vi "ShhgCommandCenter.vi"() -> ()   [LabVIEW 2015]
doc: "This template is for the Queued Message Handler design pattern.\n\nThe Event Handling Loop generates messages based on user interface actions.\n\nThe Message Handling Loop processes messages generated by the Event Handling Loop, or by other messages. The messages are string values, so new messages can be added easily to the Message Cases case structure in the Message Handling Loop. Each message cluster can also provide an optional value for Message Data, which is a variant that can be converted to whatever message-specific data is required."
uses:
  NetworkStream/NetworkStreamData.ctl
  ShhgDataLogging/DataLoggingCluster.ctl
  controls/UI Data.ctl
  DeviceLoopData.ctl
  DeviceState.ctl
  <vilib>/dex/Stream Element Allocation Mode.ctl
  <vilib>/dex/Flush And Wait Empty Condition.ctl
  <vilib>/Utility/error.llb/DialogType.ctl
  <vilib>/Utility/error.llb/Error Cluster From Error Code.vi
  support/Message Queue/Enqueue Message (Single).vi
  support/Message Queue/Enqueue Message (Array).vi
  <vilib>/ErrorRing/Error Ring.xnode
  support/Message Queue/Message Queue.lvlib
  support/User Events/User Events.lvlib
  support/Error Handling/Error Handling.lvlib
  NetworkStream/NetworkStream.lvlib
  ShhgDataLogging/ShhgDataLogging.lvlib
panel:
  out "Waiting for devices":bool
  out "Shots to go...":i32
  in  "Randomize":bool
  in  "AbortShooting":bool
  in  "Shoot":bool
  in  "RequestStatusAllDevices":bool
  in  "DisconnectAllDevices":bool
  in  "Next Shot Number":u32
  in  "Target Tabs":enum32{"Target", "Configuration"}(tab)
  out "Waiting after shot":bool
  out "Target Sequence Length (ms)":dbl=100.0
  out "Target up to date":bool
  out "Target Ready":bool
  out "Target Status":string
  out "Target Connected":bool caption="Connected"
  in  "Sequence Length (ms)":dbl=100.0
  in  "Abort Waiting after shot":bool
  in  "TargetReaderURL":string="//localhost:SolidTargetSequenceControl/SolidTargetSequenceControl"
  in  "TargetNetworkSharedVariable":refnum<k21>="ni.var.psp://localhost/SolidTargetSequenceControl/Status"
  in  "Logging Tabs":enum32{"Data Logging", "Configuration"}(tab)
  in  "DataLoggingCluster":T1={"Shot No. "=0, "Pulse Energy (mJ)"=0.0, "Pulse Duration (fs)"=0.0, "Chirp (fs^2)"=0.0, "Wedge Insertion (mm)"=0.0, "Parabola Position (um)"=0.0, "Delay (ps)"=0.0, "Seq. Length (ms)"=100.0, "Add. Param. No 1"=0.0, "Add. Param. No 2"=0.0, "Notes"=""} {"Add. Param. No 2" format="%#_6f"; "Add. Param. No 1" format="%#_6f"; "Wedge Insertion (mm)" format="%#_6f"; "Pulse Duration (fs)" format="%#_6f"; "Parabola Position (um)" format="%#_6f"; "Pulse Energy (mJ)" format="%#_6f"; "Chirp (fs^2)" format="%#_6f"}
  in  "Experiment Folder Path":path
  in  "ConnectAllDevices":bool
  out "Loop Active":bool caption="Active"
  in  "Abort Loop":bool
  in  "DelayLineTabs":enum32{"DelayLine", "Configuration"}(tab)
  out "DelayLine up to date":bool
  out "DelayLine Ready":bool
  in  "DelayLine Setpoint (ps)":dbl
  out "Delay":dbl
  out "DelayLineStatus":string
  out "DelayLineConnected":bool caption="Connected"
  in  "DelayLineReaderURL":string="//192.168.178.65/DelayLine"
  in  "DelayLineNetworkSharedVariable":refnum<k21>="ni.var.psp://pc-loa231/DelayLine/Status"
  in  "Loop End":dbl
  in  "Loop Stepsize":dbl=1.0
  in  "Loop Start":dbl
  in  "Loop Over":T2(ring)
  in  "Start Loop":bool
  in  "Exit":bool
  # "USED BY TARGET"
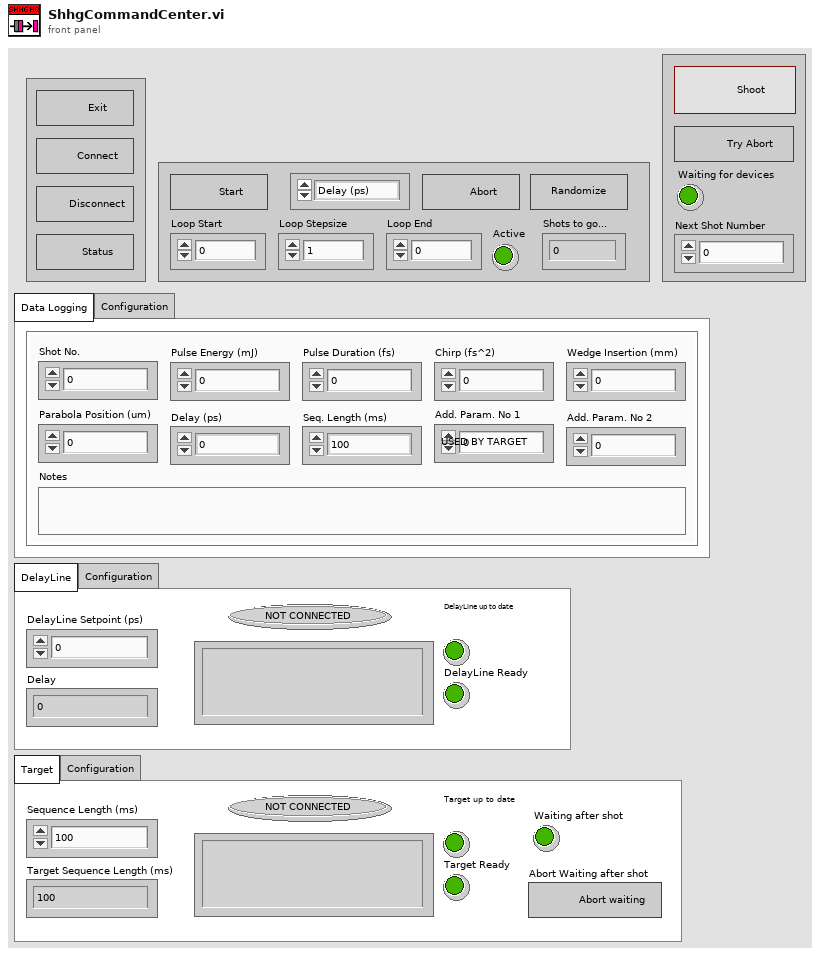
[diagram p1: front panel]
types:
  T1 = typedef "ShhgDataLogging.lvlib/DataLoggingCluster.ctl" = cluster{"Shot No. ":u32, "Pulse Energy (mJ)":dbl, "Pulse Duration (fs)":dbl, "Chirp (fs^2)":dbl, "Wedge Insertion (mm)":dbl, "Parabola Position (um)":dbl, "Delay (ps)":dbl, "Seq. Length (ms)":dbl, "Add. Param. No 1":dbl, "Add. Param. No 2":dbl, "Notes":string}
  T2 = enum16{"Delay (ps)", "Wedge (mm)", "Chirp (fs²)"}
  T3 = typedef "DeviceState.ctl" = enum16{"NotConnected", "Connected"}
  T4 = typedef "DeviceLoopData.ctl" = cluster{"shared variable refnum":refnum<k21>, "Hash":u64, "writer endpoint":refnum<k21>, "Sequence Number":u64}
  T5 = typedef "UI Data.ctl" = cluster{"Boolean <Replace Me>":bool, "String <Replace Me>":string, "Numeric <Replace Me>":dbl, "Do Something Ref":refnum<vi>, "Do Something Else Ref":refnum<vi>, "Data Display Ref":refnum<vi>, "Exit Button Ref":refnum<vi>, "LoopArray":dbl[]}
  T6 = typedef "User Events.lvlib/User Events.ctl" = cluster{"Stop":refnum<user-event>, "UserEventNo2":refnum<user-event>}
  T7 = typedef "Message Queue.lvlib/All Message Queues.ctl" = cluster{"UI":refnum<queue>, "DelayLine":refnum<queue>, "Target":refnum<queue>, "Logging":refnum<queue>}
  T8 = typedef "DialogType.ctl" = u16
  T9 = typedef "NetworkStream.lvlib/NetworkStreamData.ctl" = cluster{"Command/Status":string, "Data":variant, "Session Hash":u64, "Sequence Number":u64}
  T10 = typedef "Stream Element Allocation Mode.ctl" = u32
  T11 = typedef "Flush And Wait Empty Condition.ctl" = u8
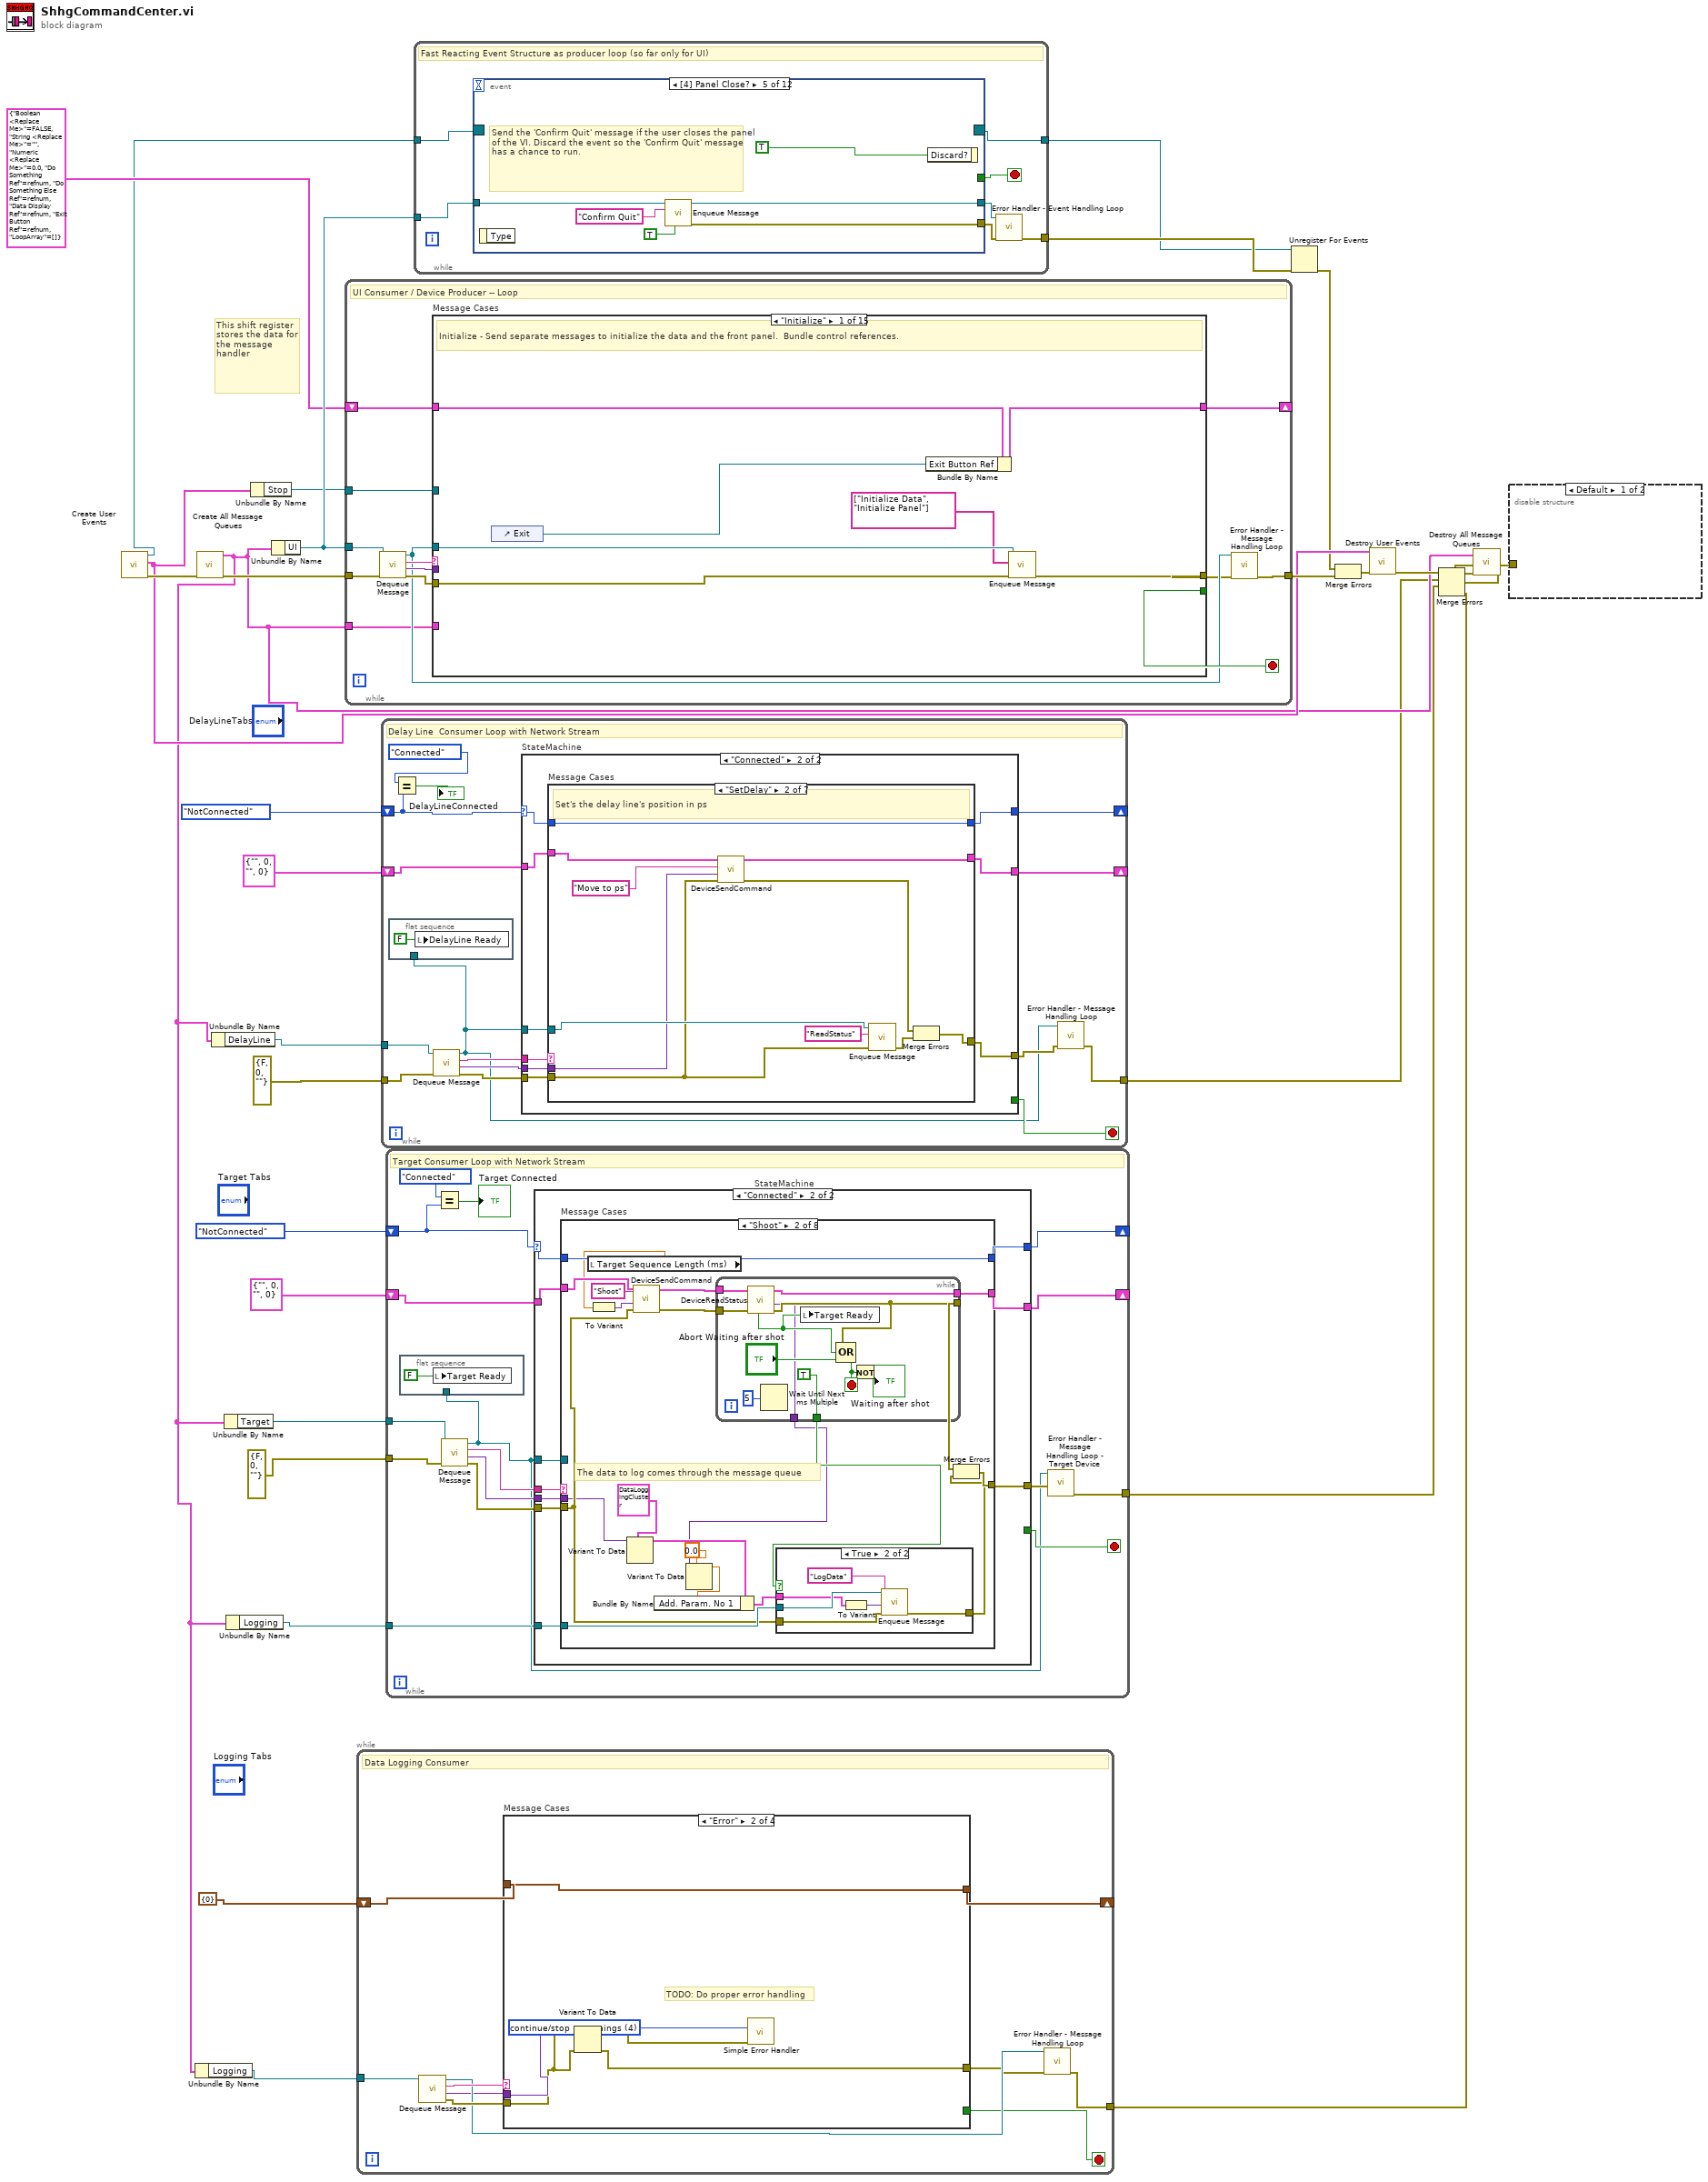
[diagram p0: block diagram]
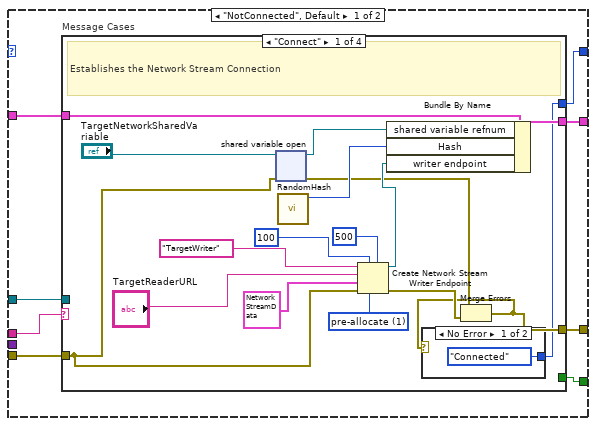
[diagram p2: hidden frame]
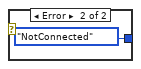
[diagram p3: hidden frame]
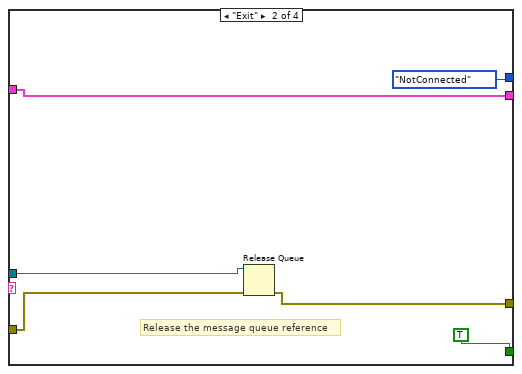
[diagram p4: hidden frame]
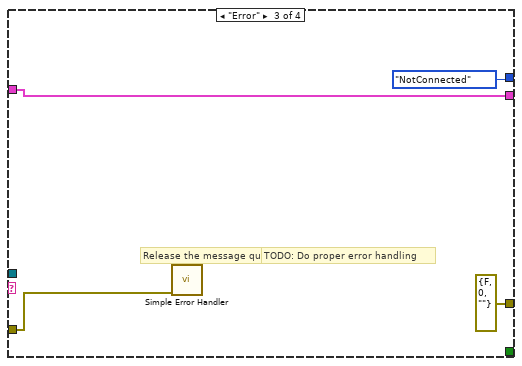
[diagram p5: hidden frame]
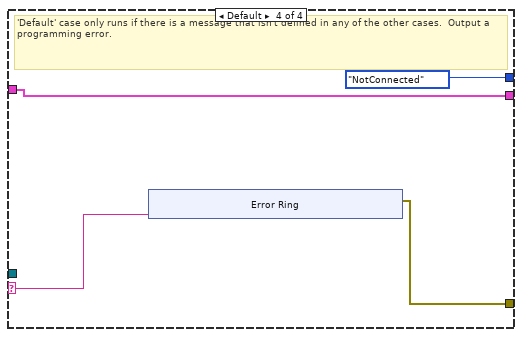
[diagram p6: hidden frame]
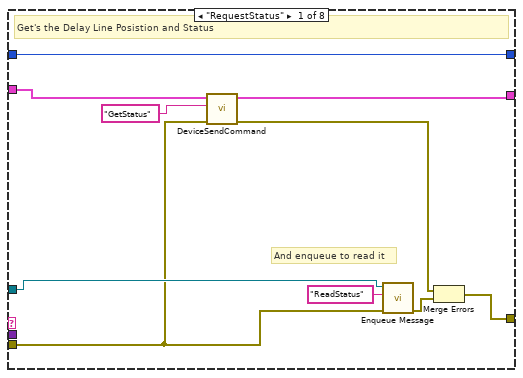
[diagram p7: hidden frame]
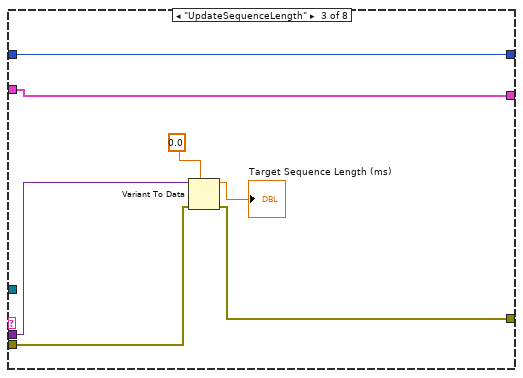
[diagram p9: hidden frame]
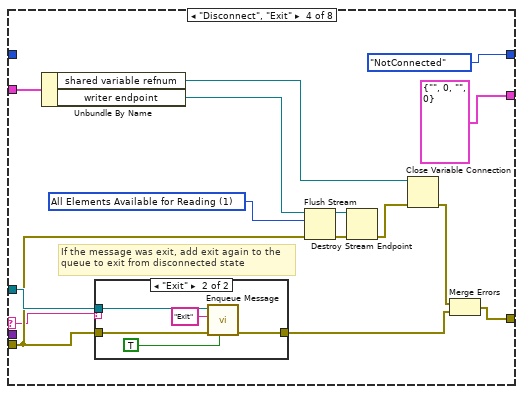
[diagram p10: hidden frame]
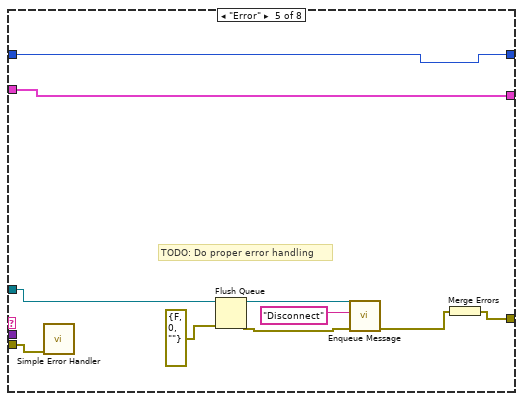
[diagram p12: hidden frame]
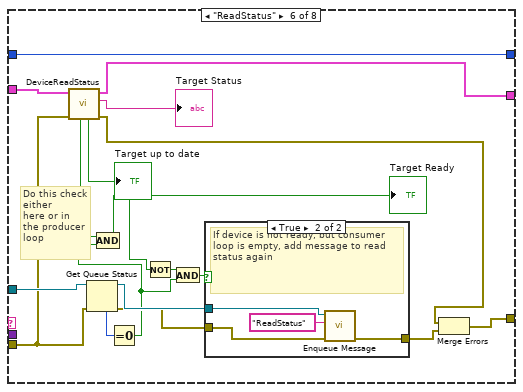
[diagram p13: hidden frame]
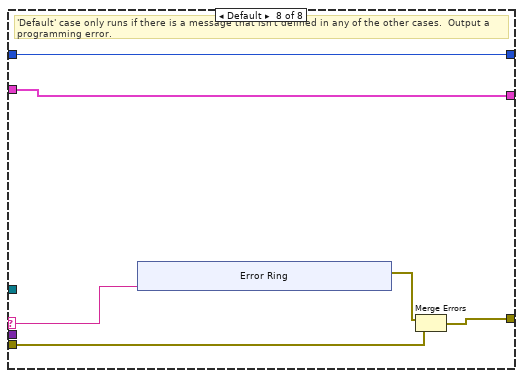
[diagram p16: hidden frame]
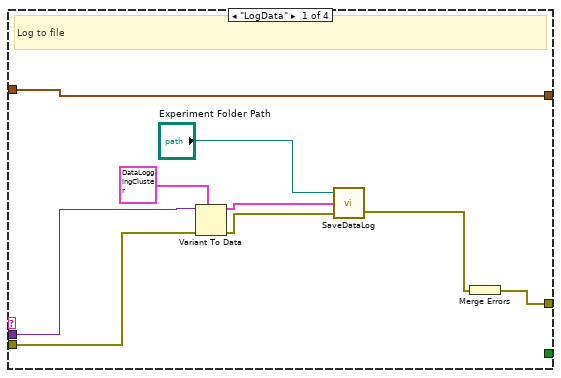
[diagram p17: hidden frame]
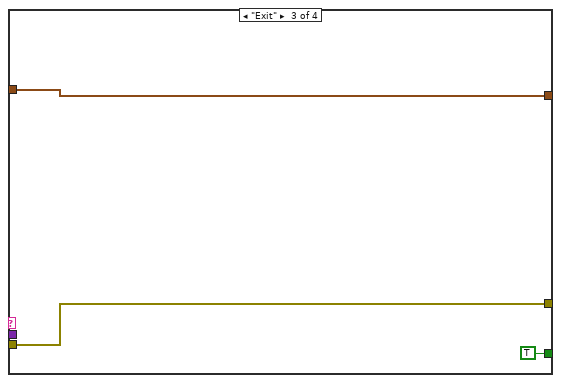
[diagram p18: hidden frame]
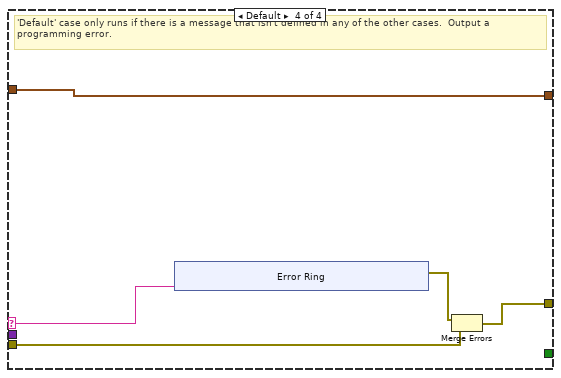
[diagram p19: hidden frame]
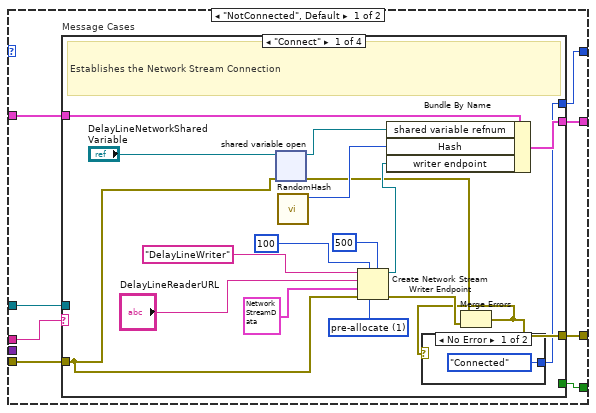
[diagram p20: hidden frame]
diagram:
  # "This shift register stores the data for the message handler"
  n1 = call "Create User Events.vi"() -> ("error out"=w27:errorcluster, "User Events"=w25:T6, "User Events Registration Refnum"=w16:refnum<event-registration>)  [unwired: 9 in]
  n2 = call "Create All Message Queues.vi"("error in (no error)"=w27) -> ("error out"=w30:errorcluster, "Message Queues out"=w6:T7)  [unwired: 9 in]
  n3 = Unbundle By Name(w6) -> ("Logging"=w13:refnum<queue>)
  n4 = Unbundle By Name(w6) -> ("DelayLine"=w18:refnum<queue>)
  n5 = Unbundle By Name(w6) -> ("Target"=w12:refnum<queue>)
  n6 = Unbundle By Name(w6) -> ("Logging"=w8:refnum<queue>)
  n7 = Unbundle By Name(w25) -> ("Stop"=w14:refnum<user-event>)
  n8 = Unbundle By Name(w6) -> ("UI"=w28:refnum<queue>)
  n9 = while {
    tunnel: w28 -> [w35]
    shift-right: [w42] -> _
    shift-left: T5 {"Boolean <Replace Me>"=FALSE, "String <Replace Me>"="", "Numeric <Replace Me>"=0.0, "Do Something Ref"=refnum, "Do Something Else Ref"=refnum, "Data Display Ref"=refnum, "Exit Button Ref"=refnum, "LoopArray"=[]} ("Data Cluster") -> [w43]
    tunnel: w14 -> [w40]
    tunnel: w30 -> [w39]
    tunnel: [w33] -> w29
    tunnel: w6 -> [w31]
    stop <- w41 stop-if-true
    # "UI Consumer / Device Producer -- Loop"
    n10 = call "Dequeue Message.vi"("error in (no error)"=w39, "Message Queue"=w35) -> ("error out"=w38:errorcluster, "Message Data"=w36:variant, "Message"=w37:string, "dup Message Queue"=w34:refnum<queue>)  [unwired: 6 in]
    n11 = case "Message Cases" shown="\"Initialize\"" w37 {
      selector: w37 -> [_ _ _ _ _ w95 _ _ _ _ _ _ _ _ w254]
      tunnel: w34 -> [w48 _ w57 w69 w81 _ _ w136 w154 _ _ _ _ w253 _]
      tunnel: w38 -> [w49 w55 w58 w77 w85 w97 w110 w138 w152 w205 w215 w225 w235 w246 _]
      tunnel: [w50 w51 w59 w70 w83 w98 w107 w137 w150 w202 w216 w226 w236 w249 w255] -> w32
      tunnel: w43 -> [w47 w54 w60 w76 w84 w99 w116 w145 w153 w207 w217 w227 w237 w252 w256]
      tunnel: [w46 w53 w60 w76 w84 w99 w116 w144 w155 w207 w217 w227 w237 w252 w256] -> w42
      tunnel: [_ _ _ _ _ _ _ _ _ _ _ _ _ TRUE _] -> w41
      tunnel: w36 -> [_ _ _ w75 _ w96 _ _ _ w200 _ _ _ _ _]
      tunnel: w40 -> [_ _ _ _ _ _ _ _ _ _ _ _ _ w248 _]
      tunnel: w31 -> [_ _ _ _ _ w93 w115 _ w151 w204 w210 w220 w230 w242 _]
      frame "Initialize" {
        # "Initialize - Send separate messages to initialize the data and the front panel.  Bundle control references."
        n12 = control-ref of="Exit"() -> (w45:refnum<vi>)
        n13 = Bundle By Name(cluster=w47, "Exit Button Ref"=w45) -> (w46:T5)
        n14 = call-poly "Enqueue Message.vi"("error in (no error)"=w49, "Message Array"=string[] ["Initialize Data", "Initialize Panel"], "Message Queue"=w48) -> ("error out"=w50:errorcluster)  [unwired: 7 in, 1 out]
      }
      frame "Initialize Data" {
        # "#CodeNeeded - Initialize your state data here."
        # "Initialize Data - Initialize the state data cluster."
        n15 = Bundle By Name(cluster=w54, "String <Replace Me>"="Initial Message" ("Initial Message")) -> (w53:T5)
        n16 = Merge Errors(w55) -> (w51:errorcluster)
      }
      frame "Initialize Panel" {
        # "Initialize Panel - Initialize the appearance of the front panel here."
        n17 = disable-structure shown="Disabled" {
          disable-tunnel: w60 -> [w66 _]
          disable-tunnel: w58 -> [w65 _]
          disable-tunnel: w57 -> [w64 _]
          disable-tunnel: [w63 _] -> w56
          frame Disabled {
            # "Send string to \"Update Display\" message"
            # "#CodeNeeded - Initialize the appearance of the front panel"
            n18 = Unbundle By Name(w66) -> ("String <Replace Me>"=w61:string)
            n19 = call-poly "Enqueue Message.vi"("error in (no error)"=w65, "Message Data"=w61, "Message"="Update Display", "Message Queue"=w64) -> ("error out"=w63:errorcluster)  [unwired: 6 in, 1 out]
          }
          frame Enabled {
          }
        }
        n20 = Merge Errors(w56) -> (w59:errorcluster)
      }
      frame "Error" {
        # "#CodeRecommended - If you ever change the name of this \"Error\" message, you'll need to update the name in the Check Loop Error.vi as well."
        # "#CodeRecommended - This code will always pop up an error dialog and call the 'Exit' message if an error occurs. Add more fine-grained error handling here."
        # "Error - Check the error message data and respond accordingly. This message is sent by the \"Error Handler\" VIs at the end of each loop in this application."
        n21 = Variant To Data(error in=w77, type=errorcluster {"status"=FALSE, "code"=0, "source"=""} ("error constant"), Variant=w75) -> (data=w73:errorcluster, error out=w72:errorcluster)
        n22 = call <vilib>:"Simple Error Handler.vi"("error in (no error)"=w73) -> ()  [unwired: 4 in, 5 out]
        n23 = call-poly "Enqueue Message.vi"("Priority Message? (F)"=TRUE, "Message"="Exit", "Message Queue"=w69) -> ("error out"=w71:errorcluster)  [unwired: 7 in, 1 out]
        n24 = Merge Errors(w71, w72) -> (w70:errorcluster)
      }
      frame "Confirm Quit" {
        # "#CodeNeeded - If you want to provide an \"Are you sure\" dialog (or some other notification) before the application exits, place that code here. This message is typically sent from a Panel Close? event."
        # "Confirm Quit - Message that can confirm whether or not the user wants to exit the application."
        n25 = Two Button Dialog(message="Do you really want to quit?", 2:"Yes!" ("T button name (\"OK\")")) -> (T button?=w78:bool)  [unwired: 1 in]
        n26 = case shown="False" w78 {
          tunnel: w85 -> [w86 w91]
          tunnel: [w86 w90] -> w82
          tunnel: w81 -> [_ w89]
          frame False {
          }
          frame True {
            n27 = call-poly "Enqueue Message.vi"("Priority Message? (F)"=TRUE, "error in (no error)"=w91, "Message"="Exit", "Message Queue"=w89) -> ("error out"=w90:errorcluster)  [unwired: 6 in, 1 out]
          }
        }
        n28 = Merge Errors(w82) -> (w83:errorcluster)
      }
      frame "SetDelay" {
        # "Duplicate this frame when creating new messages.  Change this comment in the duplicated frame to describe this message."
        n29 = Unbundle By Name(w93) -> ("DelayLine"=w92:refnum<queue>)
        n30 = call-poly "Enqueue Message.vi"("error in (no error)"=w97, "Message Data"=w96, "Message"=w95, "Message Queue"=w92) -> ("error out"=w94:errorcluster)  [unwired: 6 in, 1 out]
        n31 = Merge Errors(w94) -> (w98:errorcluster)
      }
      frame "Shoot" {
        # "Actually if the last status was ready, there should be no reason why they are not ready anmore."
        # "wait some time for target to get busy, TODO: or wait for 'Target Ready' variable to turn false"
        n32 = Unbundle By Name(w115) -> ("DelayLine"=w112:refnum<queue>, "Target"=w111:refnum<queue>)
        n33 = Increment(x="Next Shot Number") -> (x+1=w114:u32)
        n34 = local write "Next Shot Number"(w114) -> ()
        n35 = call-poly "Enqueue Message.vi"("error in (no error)"=w110, "Message"="RequestStatus", "Message Queue"=w112) -> ("error out"=w103:errorcluster)  [unwired: 7 in, 1 out]
        n36 = call-poly "Enqueue Message.vi"("error in (no error)"=w103, "Message"="RequestStatus", "Message Queue"=w111) -> ("error out"=w102:errorcluster, "dup Message Queue"=w109:refnum<queue>)  [unwired: 7 in]
        n37 = property on="Shot No." class="DigNum (strict)"(error in=w102, "Value"="Next Shot Number") -> (error out=w101:errorcluster)  [unwired: 1 in, 1 out]
        n38 = while {
          tunnel: ["AbortShooting"] -> w108
          tunnel: [w126] -> w100
          tunnel: w101 -> [w126]
          stop <- w128 stop-if-true
          n39 = local read "DelayLine Ready"() -> (w133:bool)
          n40 = local read "Target Ready"() -> (w132:bool)
          n41 = And(x=w133, y=w132) -> (x .and. y?=w131:bool)
          n42 = Or(x=w131, y="AbortShooting") -> (x .or. y?=w128:bool)
          n43 = Not(x=w128) -> (.not. x?=→"Waiting for devices":bool)
          n44 = Wait Until Next ms Multiple(millisecond multiple=u32 5) -> ()  [unwired: 1 out]
        }
        n45 = case shown="False" w108 {
          tunnel: [w120 w125] -> w107
          tunnel: w109 -> [w122 _]
          tunnel: w100 -> [w121 w125]
          tunnel: [200 0] -> w106
          frame False {
            n46 = To Variant(anything="DataLoggingCluster") -> (Variant=w118:variant)
            n47 = call-poly "Enqueue Message.vi"("error in (no error)"=w121, "Message Data"=w118, "Message"="Shoot", "Message Queue"=w122) -> ("error out"=w120:errorcluster)  [unwired: 6 in, 1 out]
          }
          frame True {
          }
        }
        n48 = Wait (ms)(milliseconds to wait=w106) -> ()  [unwired: 1 out]
      }
      frame "Start Loop" {
        # "This just generates the loop array and then dispatches the continue loop message"
        n49 = call-poly "Enqueue Message.vi"("error in (no error)"=w138, "Message"="Continue Loop", "Message Queue"=w136) -> ("error out"=w137:errorcluster)  [unwired: 7 in, 1 out]
        n50 = call "CreateLoopArray.vi"("Randomize"="Randomize", "Loop Stepsize"="Loop Stepsize", "Loop End"="Loop End", "Loop Start"="Loop Start") -> ("Loop Array"=w143:dbl[])  [unwired: 7 in]
        n51 = Bundle By Name(cluster=w145, "LoopArray"=w143) -> (w144:T5)
        n52 = local write "Loop Active"(TRUE ("Loop Active")) -> ()
      }
      frame "Continue Loop" {
        # "This just generates the loop array and then dispatches the continue loop message"
        n53 = Unbundle By Name(w153) -> ("LoopArray"=w149:dbl[])
        n54 = Array Size(array=w149) -> (size(s)=w147:i32)
        "Shots to go..." <- w147
        n55 = Not Equal To 0?(x=w147) -> (x != 0?=w148:bool)
        n56 = case shown="True" w148 {
          tunnel: [w158 w173] -> w155
          tunnel: w154 -> [_ w172]
          tunnel: w153 -> [w158 w171]
          tunnel: w149 -> [_ w170]
          tunnel: w152 -> [w156 w167]
          tunnel: w151 -> [_ w165]
          tunnel: [w156 w162] -> w150
          tunnel: [FALSE w159] -> w146
          frame False {
          }
          frame True {
            n57 = while "Wait for the target to finish shooting" {
              tunnel: ["Abort Loop"] -> w160
              tunnel: w167 -> [w193]
              tunnel: [w193] -> w164
              stop <- w195 stop-if-true
              n58 = local read "Target Ready"() -> (w196:bool)
              n59 = Or(x="Abort Loop", y=w196) -> (x .or. y?=w195:bool)
              n60 = Wait Until Next ms Multiple(millisecond multiple=u32 5) -> ()  [unwired: 1 out]
            }
            n61 = Delete From Array(array=w170, index=0) -> (deleted portion=w163:dbl, array with subset deleted=w169:dbl[])  [unwired: 1 in]
            n62 = case "Set the parameter" shown="\"Delay (ps)\", Default" "Loop Over" {
              tunnel: w165 -> [w189 _]
              tunnel: w164 -> [w190 w191]
              tunnel: w163 -> [w187 _]
              tunnel: [w184 w191] -> w161
              frame "Delay (ps)", Default {
                n63 = Unbundle By Name(w189) -> ("DelayLine"=w188:refnum<queue>)
                n64 = To Variant(anything=w187) -> (Variant=w186:variant)
                n65 = call-poly "Enqueue Message.vi"("error in (no error)"=w190, "Message Data"=w186, "Message"="SetDelay", "Message Queue"=w188) -> ("error out"=w184:errorcluster)  [unwired: 6 in, 1 out]
              }
              frame "Wedge (mm)" {
              }
            }
            n66 = Bundle By Name(cluster=w171, "LoopArray"=w169) -> (w173:T5)
            n67 = case "Enqueue continuation" shown="True" w160 {
              tunnel: w172 -> [w181 _]
              tunnel: [w177 w183] -> w162
              tunnel: w161 -> [w175 w183]
              tunnel: [TRUE FALSE] -> w159
              frame False {
                n68 = call-poly "Enqueue Message.vi"("error in (no error)"=w175, "Message"="Shoot", "Message Queue"=w181) -> ("error out"=w179:errorcluster, "dup Message Queue"=w178:refnum<queue>)  [unwired: 7 in]
                n69 = call-poly "Enqueue Message.vi"("error in (no error)"=w179, "Message"="Continue Loop", "Message Queue"=w178) -> ("error out"=w177:errorcluster)  [unwired: 7 in, 1 out]
              }
              frame True {
              }
            }
          }
        }
        "Loop Active" <- w146
      }
      frame "UpdateSequenceLength" {
        n70 = Unbundle By Name(w204) -> ("Target"=w203:refnum<queue>)
        n71 = call-poly "Enqueue Message.vi"("error in (no error)"=w205, "Message Data"=w200, "Message"="UpdateSequenceLength", "Message Queue"=w203) -> ("error out"=w198:errorcluster)  [unwired: 6 in, 1 out]
        n72 = Variant To Data(error in=w198, type=0.0 ("Value"), Variant=w200) -> (data=w199:dbl, error out=w197:errorcluster)
        n73 = property on="Seq. Length (ms)" class="DigNum (strict)"(error in=w197, "Value"=w199) -> (error out=w202:errorcluster)  [unwired: 1 in, 1 out]
      }
      frame "ConnectAllDevices" {
        # "Duplicate this frame when creating new messages.  Change this comment in the duplicated frame to describe this message."
        n74 = Unbundle By Name(w210) -> ("DelayLine"=w209:refnum<queue>, "Target"=w208:refnum<queue>)
        n75 = call-poly "Enqueue Message.vi"("error in (no error)"=w215, "Message"="Connect", "Message Queue"=w208) -> ("error out"=w211:errorcluster)  [unwired: 7 in, 1 out]
        n76 = call-poly "Enqueue Message.vi"("error in (no error)"=w211, "Message"="Connect", "Message Queue"=w209) -> ("error out"=w212:errorcluster)  [unwired: 7 in, 1 out]
        n77 = Merge Errors(w212) -> (w216:errorcluster)
      }
      frame "DisconnectAllDevices" {
        # "Duplicate this frame when creating new messages.  Change this comment in the duplicated frame to describe this message."
        n78 = Unbundle By Name(w220) -> ("DelayLine"=w219:refnum<queue>, "Target"=w218:refnum<queue>)
        n79 = call-poly "Enqueue Message.vi"("error in (no error)"=w225, "Message"="Disconnect", "Message Queue"=w218) -> ("error out"=w221:errorcluster)  [unwired: 7 in, 1 out]
        n80 = call-poly "Enqueue Message.vi"("error in (no error)"=w221, "Message"="Disconnect", "Message Queue"=w219) -> ("error out"=w222:errorcluster)  [unwired: 7 in, 1 out]
        n81 = Merge Errors(w222) -> (w226:errorcluster)
      }
      frame "RequestStatusAllDevices" {
        # "Duplicate this frame when creating new messages.  Change this comment in the duplicated frame to describe this message."
        n82 = Unbundle By Name(w230) -> ("DelayLine"=w229:refnum<queue>, "Target"=w228:refnum<queue>)
        n83 = call-poly "Enqueue Message.vi"("error in (no error)"=w235, "Message"="RequestStatus", "Message Queue"=w228) -> ("error out"=w231:errorcluster)  [unwired: 7 in, 1 out]
        n84 = call-poly "Enqueue Message.vi"("error in (no error)"=w231, "Message"="RequestStatus", "Message Queue"=w229) -> ("error out"=w232:errorcluster)  [unwired: 7 in, 1 out]
        n85 = Merge Errors(w232) -> (w236:errorcluster)
      }
      frame "Exit" {
        w241 = "Exit" ("Message")
        w243 = TRUE ("Priority Message? (F)")
        # "Stop the VI"
        # "Release the message queue reference"
        # "#CodeNeeded - Add any required cleanup code here"
        # "Exit - Exit the application."
        n86 = Unbundle By Name(w242) -> ("DelayLine"=w240:refnum<queue>, "Logging"=w239:refnum<queue>, "Target"=w238:refnum<queue>)
        n87 = call-poly "Enqueue Message.vi"("Priority Message? (F)"=w243, "error in (no error)"=w246, "Message"=w241, "Message Queue"=w238) -> ("error out"=w245:errorcluster)  [unwired: 6 in, 1 out]
        n88 = call "Fire User Event - Stop.vi"("User Event - Stop"=w248) -> ("error out"=w247:errorcluster)  [unwired: 10 in]
        n89 = Release Queue(queue=w253, error in (no error)=w246) -> (error out=w250:errorcluster)  [unwired: 1 in, 2 out]
        n90 = call-poly "Enqueue Message.vi"("Priority Message? (F)"=w243, "error in (no error)"=w245, "Message"=w241, "Message Queue"=w239) -> ("error out"=w244:errorcluster)  [unwired: 6 in, 1 out]
        n91 = call-poly "Enqueue Message.vi"("Message"=w241, "Message Queue"=w240) -> ()  [unwired: 8 in, 2 out]
        n92 = Merge Errors(w247, w250, w244) -> (w249:errorcluster)
      }
      frame Default {
        # "'Default' case only runs if there is a message that isn't defined in any of the other cases.  Output a programming error."
        n93 = xnode "Error Ring"("parameter 0"=w254) -> ("error out"=w255:errorcluster)
      }
    }
    n94 = call "Error Handler - Message Handling Loop.vi"("error in (no error)"=w32, "Message Queue"=w34) -> ("dup error in"=w33:errorcluster)  [unwired: 8 in, 1 out]
  }
  n95 = while {
    shift-right: [w272] -> _
    shift-left: cluster{i32} {0} -> [w271]
    tunnel: w13 -> [w265]
    tunnel: [w267] -> w1
    stop <- w264 stop-if-true
    # "Data Logging Consumer"
    n96 = call "Dequeue Message.vi"("Message Queue"=w265) -> ("error out"=w270:errorcluster, "Message Data"=w266:variant, "Message"=w273:string, "dup Message Queue"=w269:refnum<queue>)  [unwired: 7 in]
    n97 = case "Message Cases" shown="\"Error\"" w273 {
      selector: w273 -> [_ _ _ w296]
      tunnel: [w281 w288 w289 w295] -> w272
      tunnel: w271 -> [w281 w288 w289 w295]
      tunnel: w270 -> [w277 w285 w290 w294]
      tunnel: [w282 w286 w290 w293] -> w268
      tunnel: w266 -> [w280 w287 _ _]
      tunnel: [_ _ TRUE _] -> w264
      frame "LogData" {
        # "Log to file"
        n98 = Variant To Data(error in=w277, type=T1 {"Shot No. "=0, "Pulse Energy (mJ)"=0.0, "Pulse Duration (fs)"=0.0, "Chirp (fs^2)"=0.0, "Wedge Insertion (mm)"=0.0, "Parabola Position (um)"=0.0, "Delay (ps)"=0.0, "Seq. Length (ms)"=0.0, "Add. Param. No 1"=0.0, "Add. Param. No 2"=0.0, "Notes"=""} ("DataLoggingCluster"), Variant=w280) -> (data=w278:T1, error out=w275:errorcluster)
        n99 = call "SaveDataLog.vi"("entrée d'erreur"=w275, "DataLoggingCluster"=w278, "chemin du fichier (utiliser une boîte de dialogue)"="Experiment Folder Path") -> ("sortie d'erreur"=w274:errorcluster)  [unwired: 1 in]
        n100 = Merge Errors(w274) -> (w282:errorcluster)
      }
      frame "Error" {
        w283 = T8 4 items=["no dialog", "OK message", "continue or stop message", "OK message + warnings", "continue/stop + warnings"] ("type of dialog (OK msg:1)")
        # "TODO: Do proper error handling"
        n101 = Variant To Data(error in=w285, type=w285, Variant=w287) -> (data=w284:errorcluster, error out=w286:errorcluster)
        n102 = call <vilib>:"Simple Error Handler.vi"("type of dialog (OK msg:1)"=w283, "error in (no error)"=w284) -> ()  [unwired: 3 in, 5 out]
      }
      frame "Exit" {
      }
      frame Default {
        # "'Default' case only runs if there is a message that isn't defined in any of the other cases.  Output a programming error."
        n103 = xnode "Error Ring"("parameter 0"=w296) -> ("error out"=w292:errorcluster)
        n104 = Merge Errors(w292, w294) -> (w293:errorcluster)
      }
    }
    n105 = call "Error Handler - Message Handling Loop.vi"("error in (no error)"=w268, "Message Queue"=w269) -> ("dup error in"=w267:errorcluster)  [unwired: 8 in, 1 out]
  }
  n106 = while {
    shift-right: [w318] -> _
    shift-left: DeviceState."NotConnected" -> [w315]
    shift-right: [w313] -> _
    shift-left: T4 {"shared variable refnum"="", "Hash"=0, "writer endpoint"="", "Sequence Number"=0} -> [w312]
    tunnel: w18 -> [w307]
    tunnel: errorcluster {"status"=FALSE, "code"=0, "source"=""} ("error in (no error)") -> [w311]
    tunnel: [w308] -> w3
    stop <- w305 stop-if-true
    # "Delay Line  Consumer Loop with Network Stream"
    n107 = flat-sequence {
      tunnel: w304 -> [_]
      frame #0 {
        n108 = local write "DelayLine Ready"(FALSE ("DelayLine Ready")) -> ()
      }
    }
    n109 = Equal?(x=DeviceState."Connected", y=w315) -> (x = y?=→"DelayLineConnected":bool)
    n110 = call "Dequeue Message.vi"("error in (no error)"=w311, "Message Queue"=w307) -> ("error out"=w310:errorcluster, "Message Data"=w306:variant, "Message"=w317:string, "dup Message Queue"=w304:refnum<queue>)  [unwired: 6 in]
    n111 = case "StateMachine" shown="\"Connected\"" w315 {
      selector: w315 -> [_ w373]
      tunnel: [w322 w372] -> w318
      tunnel: w317 -> [w327 w375]
      tunnel: [w326 w370] -> w313
      tunnel: w312 -> [w325 w376]
      tunnel: w310 -> [w324 w374]
      tunnel: [w323 w371] -> w309
      tunnel: w304 -> [w321 w369]
      tunnel: w306 -> [_ w368]
      tunnel: [w320 _] -> w305
      frame "NotConnected", Default {
        n112 = case "Message Cases" shown="\"Connect\"" w327 {
          selector: w327 -> [_ _ _ w360]
          tunnel: [w344 w347 w355 w359] -> w326
          tunnel: w325 -> [w343 w347 w355 w359]
          tunnel: w324 -> [w333 w352 w354 _]
          tunnel: [w329 w350 errorcluster {"status"=FALSE, "code"=0, "source"=""} ("error out") w357] -> w323
          tunnel: [w328 DeviceState."NotConnected" DeviceState."NotConnected" DeviceState."NotConnected"] -> w322
          tunnel: w321 -> [_ w351 _ _]
          tunnel: [_ TRUE _ _] -> w320
          frame "Connect" {
            w337 = T10 1 items=["allocate as needed", "pre-allocate"] ("element allocation mode")
            # "Establishes the Network Stream Connection"
            n113 = shared-variable-open("DelayLineNetworkSharedVariable", w333) -> (w341:refnum<k21>, w331:errorcluster)
            n114 = call "RandomHash.vi"() -> ("Numeric Control"=w340:u64)  [unwired: 11 in]
            n115 = Create Network Stream Writer Endpoint(5:500 ("timeout in ms (-1)"), 6:w337, 7:100 ("writer buffer size"), 8:w333, 9:T9 {"Command/Status"="", "Data"=variant, "Session Hash"=0, "Sequence Number"=0} ("NetworkStreamCluster"), 10:"DelayLineReaderURL", 11:"DelayLineWriter" ("writer name")) -> (0:w330:errorcluster, 3:w332:refnum<k21>)
            n116 = Bundle By Name(cluster=w343, "shared variable refnum"=w341, "Hash"=w340, "writer endpoint"=w332) -> (w344:T4)
            n117 = Merge Errors(w331, w330) -> (w329:errorcluster)
            n118 = case shown="No Error" w329 {
              tunnel: [DeviceState."Connected" ("x") DeviceState."NotConnected"] -> w328
              frame No Error {
              }
              frame Error {
              }
            }
          }
          frame "Exit" {
            # "Release the message queue reference"
            n119 = Release Queue(queue=w351, error in (no error)=w352) -> (error out=w350:errorcluster)  [unwired: 1 in, 2 out]
          }
          frame "Error" {
            # "TODO: Do proper error handling"
            # "Release the message queue reference"
            n120 = call <vilib>:"Simple Error Handler.vi"("error in (no error)"=w354) -> ()  [unwired: 4 in, 5 out]
          }
          frame Default {
            # "'Default' case only runs if there is a message that isn't defined in any of the other cases.  Output a programming error."
            n121 = xnode "Error Ring"("parameter 0"=w360) -> ("error out"=w357:errorcluster)
          }
        }
      }
      frame "Connected" {
        n122 = case "Message Cases" shown="\"SetDelay\"" w375 {
          selector: w375 -> [_ _ w398 _ _ _ w468]
          tunnel: [w383 w394 T4 {"shared variable refnum"="", "Hash"=0, "writer endpoint"="", "Sequence Number"=0} w424 w448 w462 w467] -> w370
          tunnel: w376 -> [w385 w396 w407 w424 w449 w462 w467]
          tunnel: w374 -> [w378 w389 w401 w420 w443 w460 w465]
          tunnel: [w377 w388 w400 w428 w441 w460 w464] -> w371
          tunnel: w373 -> [w386 w397 _ w425 w445 w461 w466]
          tunnel: [w386 w397 DeviceState."NotConnected" w425 w445 w461 w466] -> w372
          tunnel: w369 -> [w381 w392 w402 w423 w444 _ _]
          tunnel: w368 -> [_ w387 _ _ _ _ _]
          frame "RequestStatus" {
            # "Get's the Delay Line Posistion and Status"
            n123 = call "DeviceSendCommand.vi"("error in (no error)"=w378, "Command/Status"="GetStatus", "DeviceLoopData"=w385) -> ("error out"=w379:errorcluster, "DeviceLoopData Out"=w383:T4)  [unwired: 7 in]
            n124 = call-poly "Enqueue Message.vi"("error in (no error)"=w378, "Message"="ReadStatus", "Message Queue"=w381) -> ("error out"=w380:errorcluster)  [unwired: 7 in, 1 out]
            n125 = Merge Errors(w379, w380) -> (w377:errorcluster)
          }
          frame "SetDelay" {
            # "Set's the delay line's position in ps"
            n126 = call "DeviceSendCommand.vi"("error in (no error)"=w389, "Data"=w387, "Command/Status"="Move to ps", "DeviceLoopData"=w396) -> ("error out"=w390:errorcluster, "DeviceLoopData Out"=w394:T4)  [unwired: 6 in]
            n127 = call-poly "Enqueue Message.vi"("error in (no error)"=w389, "Message"="ReadStatus", "Message Queue"=w392) -> ("error out"=w391:errorcluster)  [unwired: 7 in, 1 out]
            n128 = Merge Errors(w390, w391) -> (w388:errorcluster)
          }
          frame "Disconnect", "Exit" {
            w412 = T11 1 items=["All Elements Read From Stream", "All Elements Available for Reading"] ("wait condition")
            # "If the message was exit, add exit again to the\nqueue to exit from disconnected state"
            n129 = Unbundle By Name(w407) -> ("shared variable refnum"=w408:refnum<k21>, "writer endpoint"=w406:refnum<k21>)
            n130 = case shown="\"Exit\"" w398 {
              tunnel: w402 -> [_ w416]
              tunnel: w401 -> [w413 w415]
              tunnel: [w413 w414] -> w399
              frame "False", Default {
              }
              frame "Exit" {
                n131 = call-poly "Enqueue Message.vi"("Priority Message? (F)"=TRUE, "error in (no error)"=w415, "Message"="Exit", "Message Queue"=w416) -> ("error out"=w414:errorcluster)  [unwired: 6 in, 1 out]
              }
            }
            n132 = Flush Stream(8:w401, 10:w412, 11:w406) -> (0:w411:errorcluster, 3:w410:refnum<k21>)  [unwired: 1 in, 1 out]
            n133 = Destroy Stream Endpoint(8:w411, 11:w410) -> (0:w404:errorcluster)
            n134 = Close Variable Connection(8:w404, 11:w408) -> (0:w403:errorcluster)
            n135 = Merge Errors(w403, w399) -> (w400:errorcluster)
          }
          frame "Error" {
            # "TODO: Do proper error handling"
            n136 = call <vilib>:"Simple Error Handler.vi"("error in (no error)"=w420) -> ()  [unwired: 4 in, 5 out]
            n137 = Flush Queue(queue=w423, error in (no error)=errorcluster {"status"=FALSE, "code"=0, "source"=""}) -> (queue out=w422:refnum<queue>, error out=w421:errorcluster)  [unwired: 1 out]
            n138 = call-poly "Enqueue Message.vi"("error in (no error)"=w421, "Message"="Disconnect", "Message Queue"=w422) -> ("error out"=w427:errorcluster)  [unwired: 7 in, 1 out]
            n139 = Merge Errors(w427) -> (w428:errorcluster)
          }
          frame "ReadStatus" {
            # "Do this check either\nhere or in the producer loop"
            n140 = call "DeviceReadStatus.vi"("error in (no error)"=w443, "DeviceLoopData in"=w449) -> ("error out"=w450:errorcluster, "Data"=w451:variant, "Status"=→"DelayLineStatus":string, "DeviceLoopData out"=w448:T4, "Up To Date"=→"DelayLine up to date":bool, "Ready"=w440:bool)  [unwired: 4 in]
            n141 = Get Queue Status(queue=w444, error in (no error)=w443) -> (queue out=w433:refnum<queue>, error out=w434:errorcluster, # elements in queue=w442:i32)  [unwired: 1 in, 5 out]
            n142 = Equal To 0?(x=w442) -> (x = 0?=w435:bool)
            n143 = Compound Arithmetic op=AND(w440, w435) -> (w436:bool)
            n144 = Not(x=w436) -> (.not. x?=w438:bool)
            n145 = Variant To Data(error in=w450, type=0.0, Variant=w451) -> (data=w431:dbl, error out=w432:errorcluster)
            "Delay" <- w431
            n146 = And(x=w438, y=w435) -> (x .and. y?=w437:bool)
            n147 = case shown="False" w437 {
              tunnel: w433 -> [_ w459]
              tunnel: w434 -> [w455 w458]
              tunnel: [w455 w457] -> w439
              frame False {
              }
              frame True {
                # "If device is not ready, but consumer loop is empty, add message to read status again"
                n148 = call-poly "Enqueue Message.vi"("error in (no error)"=w458, "Message"="ReadStatus", "Message Queue"=w459) -> ("error out"=w457:errorcluster)  [unwired: 7 in, 1 out]
              }
            }
            n149 = property on="Delay (ps)" class="DigNum (strict)"(error in=w432, "Value"=w431) -> (error out=w430:errorcluster)  [unwired: 1 in, 1 out]
            n150 = flat-sequence {
              tunnel: w436 -> [w454]
              tunnel: w430 -> [w453]
              tunnel: [w453] -> w429
              frame #0 {
                # "Only be ready when also the data has been written"
                "DelayLine Ready" <- w454
              }
            }
            n151 = Merge Errors(w429, w439) -> (w441:errorcluster)
          }
          frame "Connect" {
            # "Nothing to do here"
          }
          frame Default {
            # "'Default' case only runs if there is a message that isn't defined in any of the other cases.  Output a programming error."
            n152 = xnode "Error Ring"("parameter 0"=w468) -> ("error out"=w463:errorcluster)
            n153 = Merge Errors(w463, w465) -> (w464:errorcluster)
          }
        }
      }
    }
    n154 = call "Error Handler - Message Handling Loop.vi"("error in (no error)"=w309, "Message Queue"=w304) -> ("dup error in"=w308:errorcluster)  [unwired: 8 in, 1 out]
  }
  n155 = while {
    tunnel: w12 -> [w491]
    tunnel: errorcluster {"status"=FALSE, "code"=0, "source"=""} ("error in (no error)") -> [w490]
    shift-right: [w479] -> _
    shift-left: T4 {"shared variable refnum"="", "Hash"=0, "writer endpoint"="", "Sequence Number"=0} -> [w486]
    shift-right: [w478] -> _
    shift-left: DeviceState."NotConnected" -> [w487]
    tunnel: w8 -> [w480]
    tunnel: [w477] -> w2
    stop <- w482 stop-if-true
    # "Target Consumer Loop with Network Stream"
    n156 = flat-sequence {
      tunnel: w476 -> [_]
      frame #0 {
        n157 = local write "Target Ready"(FALSE ("DelayLine Ready")) -> ()
      }
    }
    n158 = Equal?(x=DeviceState."Connected", y=w487) -> (x = y?=→"Target Connected":bool)
    n159 = call "Dequeue Message.vi"("error in (no error)"=w490, "Message Queue"=w491) -> ("error out"=w483:errorcluster, "Message Data"=w484:variant, "Message"=w485:string, "dup Message Queue"=w476:refnum<queue>)  [unwired: 6 in]
    n160 = case "StateMachine" shown="\"Connected\"" w487 {
      selector: w487 -> [_ w547]
      tunnel: [w495 w546] -> w478
      tunnel: w485 -> [w500 w549]
      tunnel: [w499 w544] -> w479
      tunnel: w486 -> [w498 w550]
      tunnel: w483 -> [w497 w548]
      tunnel: [w496 w545] -> w481
      tunnel: w476 -> [w494 w543]
      tunnel: w484 -> [_ w542]
      tunnel: [w493 _] -> w482
      tunnel: w480 -> [_ w541]
      frame "NotConnected", Default {
        n161 = case "Message Cases" shown="\"Connect\"" w500 {
          selector: w500 -> [_ _ _ w533]
          tunnel: [w517 w520 w528 w532] -> w499
          tunnel: w498 -> [w516 w520 w528 w532]
          tunnel: w497 -> [w508 w525 w527 _]
          tunnel: [w504 w523 errorcluster {"status"=FALSE, "code"=0, "source"=""} ("error out") w530] -> w496
          tunnel: [w503 DeviceState."NotConnected" DeviceState."NotConnected" DeviceState."NotConnected"] -> w495
          tunnel: w494 -> [_ w524 _ _]
          tunnel: [_ TRUE _ _] -> w493
          frame "Connect" {
            w511 = T10 1 items=["allocate as needed", "pre-allocate"] ("element allocation mode")
            # "Establishes the Network Stream Connection"
            n162 = shared-variable-open("TargetNetworkSharedVariable", w508) -> (w515:refnum<k21>, w506:errorcluster)
            n163 = call "RandomHash.vi"() -> ("Numeric Control"=w514:u64)  [unwired: 11 in]
            n164 = Create Network Stream Writer Endpoint(5:500 ("timeout in ms (-1)"), 6:w511, 7:100 ("writer buffer size"), 8:w508, 9:T9 {"Command/Status"="", "Data"=variant, "Session Hash"=0, "Sequence Number"=0} ("NetworkStreamCluster"), 10:"TargetReaderURL", 11:"TargetWriter" ("writer name")) -> (0:w505:errorcluster, 3:w507:refnum<k21>)
            n165 = Bundle By Name(cluster=w516, "shared variable refnum"=w515, "Hash"=w514, "writer endpoint"=w507) -> (w517:T4)
            n166 = Merge Errors(w506, w505) -> (w504:errorcluster)
            n167 = case shown="No Error" w504 {
              tunnel: [DeviceState."Connected" ("x") DeviceState."NotConnected"] -> w503
              frame No Error {
              }
              frame Error {
              }
            }
          }
          frame "Exit" {
            # "Release the message queue reference"
            n168 = Release Queue(queue=w524, error in (no error)=w525) -> (error out=w523:errorcluster)  [unwired: 1 in, 2 out]
          }
          frame "Error" {
            # "TODO: Do proper error handling"
            # "Release the message queue reference"
            n169 = call <vilib>:"Simple Error Handler.vi"("error in (no error)"=w527) -> ()  [unwired: 4 in, 5 out]
          }
          frame Default {
            # "'Default' case only runs if there is a message that isn't defined in any of the other cases.  Output a programming error."
            n170 = xnode "Error Ring"("parameter 0"=w533) -> ("error out"=w530:errorcluster)
          }
        }
      }
      frame "Connected" {
        n171 = case "Message Cases" shown="\"Shoot\"" w549 {
          selector: w549 -> [_ _ _ w607 _ _ _ w669]
          tunnel: [w557 w570 w605 T4 {"shared variable refnum"="", "Hash"=0, "writer endpoint"="", "Sequence Number"=0} w633 w654 w662 w668] -> w544
          tunnel: w550 -> [w559 w577 w605 w616 w633 w655 w662 w668]
          tunnel: w548 -> [w552 w574 w601 w610 w629 w651 w661 w666]
          tunnel: [w551 w581 w600 w609 w637 w647 w661 w665] -> w545
          tunnel: w547 -> [w560 w578 w606 _ w634 w653 w663 w667]
          tunnel: [w560 w578 w606 DeviceState."NotConnected" w634 w653 w663 w667] -> w546
          tunnel: w543 -> [w555 _ _ w611 w632 w652 _ _]
          tunnel: w542 -> [_ w567 w602 _ _ _ _ _]
          tunnel: w541 -> [_ w579 _ _ _ _ _ _]
          frame "RequestStatus" {
            # "And enqueue to read it"
            # "Get's the Delay Line Posistion and Status"
            n172 = call "DeviceSendCommand.vi"("error in (no error)"=w552, "Command/Status"="GetStatus", "DeviceLoopData"=w559) -> ("error out"=w553:errorcluster, "DeviceLoopData Out"=w557:T4)  [unwired: 7 in]
            n173 = call-poly "Enqueue Message.vi"("error in (no error)"=w552, "Message"="ReadStatus", "Message Queue"=w555) -> ("error out"=w554:errorcluster)  [unwired: 7 in, 1 out]
            n174 = Merge Errors(w553, w554) -> (w551:errorcluster)
          }
          frame "Shoot" {
            # "The data to log comes through the message queue"
            n175 = local read "Target Sequence Length (ms)"() -> (w575:dbl)
            n176 = To Variant(anything=w575) -> (Variant=w576:variant)
            n177 = Variant To Data(type=T1 {"Shot No. "=0, "Pulse Energy (mJ)"=0.0, "Pulse Duration (fs)"=0.0, "Chirp (fs^2)"=0.0, "Wedge Insertion (mm)"=0.0, "Parabola Position (um)"=0.0, "Delay (ps)"=0.0, "Seq. Length (ms)"=0.0, "Add. Param. No 1"=0.0, "Add. Param. No 2"=0.0, "Notes"=""} ("DataLoggingCluster 2"), Variant=w567) -> (data=w566:T1)  [unwired: 1 in, 1 out]
            n178 = call "DeviceSendCommand.vi"("error in (no error)"=w574, "Data"=w576, "Command/Status"="Shoot", "DeviceLoopData"=w577) -> ("error out"=w572:errorcluster, "DeviceLoopData Out"=w571:T4)  [unwired: 6 in]
            n179 = while {
              tunnel: w572 -> [w592]
              tunnel: w571 -> [w591]
              tunnel: [w589] -> w570
              tunnel: [TRUE] -> w569
              tunnel: [w585] -> w568
              tunnel: [w582] -> w563
              stop <- w584 stop-if-true
              n180 = call "DeviceReadStatus.vi"("error in (no error)"=w592, "DeviceLoopData in"=w591) -> ("error out"=w585:errorcluster, "Data"=w582:variant, "DeviceLoopData out"=w589:T4, "Ready"=w587:bool)  [unwired: 4 in, 2 out]
              n181 = Wait Until Next ms Multiple(millisecond multiple=u32 5) -> ()  [unwired: 1 out]
              n182 = local write "Target Ready"(w587) -> ()
              n183 = Compound Arithmetic op=OR(w585, w587, "Abort Waiting after shot") -> (w584:bool)
              n184 = Not(x=w584) -> (.not. x?=→"Waiting after shot":bool)
            }
            n185 = Variant To Data(type=0.0 ("Add. Param. No 1"), Variant=w563) -> (data=w562:dbl)  [unwired: 1 in, 1 out]
            n186 = Bundle By Name(cluster=w566, "Add. Param. No 1"=w562) -> (w564:T1)
            n187 = case shown="True" w569 {
              tunnel: w574 -> [w593 w599]
              tunnel: [w593 w598] -> w580
              tunnel: w579 -> [_ w597]
              tunnel: w564 -> [_ w594]
              frame False {
              }
              frame True {
                n188 = To Variant(anything=w594) -> (Variant=w596:variant)
                n189 = call-poly "Enqueue Message.vi"("error in (no error)"=w599, "Message Data"=w596, "Message"="LogData", "Message Queue"=w597) -> ("error out"=w598:errorcluster)  [unwired: 6 in, 1 out]
              }
            }
            n190 = Merge Errors(w568, w580) -> (w581:errorcluster)
          }
          frame "UpdateSequenceLength" {
            n191 = Variant To Data(error in=w601, type=0.0 ("Target Sequence Length (ms) 2"), Variant=w602) -> (data=→"Target Sequence Length (ms)":dbl, error out=w600:errorcluster)
          }
          frame "Disconnect", "Exit" {
            w621 = T11 1 items=["All Elements Read From Stream", "All Elements Available for Reading"] ("wait condition")
            # "If the message was exit, add exit again to the\nqueue to exit from disconnected state"
            n192 = Unbundle By Name(w616) -> ("shared variable refnum"=w617:refnum<k21>, "writer endpoint"=w615:refnum<k21>)
            n193 = case shown="\"Exit\"" w607 {
              tunnel: w611 -> [_ w625]
              tunnel: w610 -> [w622 w624]
              tunnel: [w622 w623] -> w608
              frame "False", Default {
              }
              frame "Exit" {
                n194 = call-poly "Enqueue Message.vi"("Priority Message? (F)"=TRUE, "error in (no error)"=w624, "Message"="Exit", "Message Queue"=w625) -> ("error out"=w623:errorcluster)  [unwired: 6 in, 1 out]
              }
            }
            n195 = Flush Stream(8:w610, 10:w621, 11:w615) -> (0:w620:errorcluster, 3:w619:refnum<k21>)  [unwired: 1 in, 1 out]
            n196 = Destroy Stream Endpoint(8:w620, 11:w619) -> (0:w613:errorcluster)
            n197 = Close Variable Connection(8:w613, 11:w617) -> (0:w612:errorcluster)
            n198 = Merge Errors(w612, w608) -> (w609:errorcluster)
          }
          frame "Error" {
            # "TODO: Do proper error handling"
            n199 = call <vilib>:"Simple Error Handler.vi"("error in (no error)"=w629) -> ()  [unwired: 4 in, 5 out]
            n200 = Flush Queue(queue=w632, error in (no error)=errorcluster {"status"=FALSE, "code"=0, "source"=""}) -> (queue out=w631:refnum<queue>, error out=w630:errorcluster)  [unwired: 1 out]
            n201 = call-poly "Enqueue Message.vi"("error in (no error)"=w630, "Message"="Disconnect", "Message Queue"=w631) -> ("error out"=w636:errorcluster)  [unwired: 7 in, 1 out]
            n202 = Merge Errors(w636) -> (w637:errorcluster)
          }
          frame "ReadStatus" {
            # "Do this check either\nhere or in the producer loop"
            n203 = call "DeviceReadStatus.vi"("error in (no error)"=w651, "DeviceLoopData in"=w655) -> ("error out"=w645:errorcluster, "Status"=→"Target Status":string, "DeviceLoopData out"=w654:T4, "Up To Date"=→"Target up to date":bool, "Ready"=w642:bool)  [unwired: 4 in, 1 out]
            n204 = Get Queue Status(queue=w652, error in (no error)=w651) -> (queue out=w649:refnum<queue>, error out=w648:errorcluster, # elements in queue=w650:i32)  [unwired: 1 in, 5 out]
            n205 = Equal To 0?(x=w650) -> (x = 0?=w640:bool)
            n206 = Compound Arithmetic op=AND(w642, w640) -> (w638:bool)
            "Target Ready" <- w638
            n207 = Not(x=w638) -> (.not. x?=w639:bool)
            n208 = And(x=w639, y=w640) -> (x .and. y?=w641:bool)
            n209 = case shown="True" w641 {
              tunnel: w649 -> [_ w660]
              tunnel: w648 -> [w656 w659]
              tunnel: [w656 w658] -> w646
              frame False {
              }
              frame True {
                # "If device is not ready, but consumer loop is empty, add message to read status again"
                n210 = call-poly "Enqueue Message.vi"("error in (no error)"=w659, "Message"="ReadStatus", "Message Queue"=w660) -> ("error out"=w658:errorcluster)  [unwired: 7 in, 1 out]
              }
            }
            n211 = Merge Errors(w645, w646) -> (w647:errorcluster)
          }
          frame "Connect" {
            # "Nothing to do here, we are already connected"
          }
          frame Default {
            # "'Default' case only runs if there is a message that isn't defined in any of the other cases.  Output a programming error."
            n212 = xnode "Error Ring"("parameter 0"=w669) -> ("error out"=w664:errorcluster)
            n213 = Merge Errors(w664, w666) -> (w665:errorcluster)
          }
        }
      }
    }
    n214 = call "Error Handler - Message Handling Loop - Target Device.vi"("error in (no error)"=w481, "Message Queue"=w476) -> ("dup error in"=w477:errorcluster)  [unwired: 8 in, 1 out]
  }
  n215 = while {
    tunnel: w28 -> [w683]
    tunnel: [w679] -> w22
    tunnel: w16 -> [w678]
    tunnel: [w677] -> w15
    stop <- w681 stop-if-true
    # "Fast Reacting Event Structure as producer loop (so far only for UI)"
    n216 = event shown="[4] Panel Close?" {
      selector: w678 -> [_ _ _ _ _ _ _ _ _ _ _ _]
      dyn-events: [_ _ _ _ _ _ _ _ _ _ _ _] -> w677
      timeout: _ -> [_ _ _ _ _ _ _ _ _ _ _ _]
      tunnel: [_ _ _ _ _ TRUE ("Discard?") _ _ _ _ TRUE ("Discard?") _] -> w681
      tunnel: w683 -> [w687 w691 w695 w701 w706 w710 w715 w719 w723 w729 w732 w734]
      tunnel: [w684 w688 w692 w698 w705 errorcluster {"status"=FALSE, "code"=0, "source"=""} ("error out") w714 w716 w720 w726 errorcluster {"status"=FALSE, "code"=0, "source"=""} ("error out") errorcluster {"status"=FALSE, "code"=0, "source"=""} ("error out")] -> w682
      tunnel: [w686 w690 w694 w700 w704 w710 w713 w718 w722 w728 w732 w734] -> w680
      event "ConnectAllDevices": Value Change {
        n217 = event-data() -> ()  [unwired: 1 in, 1 out]
        n218 = call-poly "Enqueue Message.vi"("Message"="ConnectAllDevices", "Message Queue"=w687) -> ("error out"=w684:errorcluster, "dup Message Queue"=w686:refnum<queue>)  [unwired: 8 in]
      }
      event "DisconnectAllDevices": Value Change {
        n219 = event-data() -> ()  [unwired: 1 in, 1 out]
        n220 = call-poly "Enqueue Message.vi"("Message"="DisconnectAllDevices", "Message Queue"=w691) -> ("error out"=w688:errorcluster, "dup Message Queue"=w690:refnum<queue>)  [unwired: 8 in]
      }
      event "RequestStatusAllDevices": Value Change {
        n221 = event-data() -> ()  [unwired: 1 in, 1 out]
        n222 = call-poly "Enqueue Message.vi"("Message"="RequestStatusAllDevices", "Message Queue"=w695) -> ("error out"=w692:errorcluster, "dup Message Queue"=w694:refnum<queue>)  [unwired: 8 in]
      }
      event "DelayLine Setpoint (ps)": Value Change {
        n223 = event-data() -> ()  [unwired: 1 in, 1 out]
        n224 = To Variant(anything="DelayLine Setpoint (ps)") -> (Variant=w696:variant)
        n225 = call-poly "Enqueue Message.vi"("Message Data"=w696, "Message"="SetDelay", "Message Queue"=w701) -> ("error out"=w698:errorcluster, "dup Message Queue"=w700:refnum<queue>)  [unwired: 7 in]
      }
      event Panel Close? {
        # "Send the 'Confirm Quit' message if the user closes the panel of the VI. Discard the event so the 'Confirm Quit' message has a chance to run."
        n226 = event-data() -> ()  [unwired: 1 in, 1 out]
        n227 = call-poly "Enqueue Message.vi"("Priority Message? (F)"=TRUE, "Message"="Confirm Quit", "Message Queue"=w706) -> ("error out"=w705:errorcluster, "dup Message Queue"=w704:refnum<queue>)  [unwired: 7 in]
        n228 = event-data("Discard?"=TRUE) -> ()  [unwired: 1 in, 1 out]
      }
      event Application Instance Close {
        # "#CodeRecommended - When a project closes, all VIs within that project are aborted and leave memory. However, any code placed in this event frame is guaranteed to run to completion, so add any cleanup code that absolutely must happen here."
        n229 = event-data() -> ()  [unwired: 1 in, 1 out]
      }
      event "Exit": Value Change {
        n230 = event-data() -> ()  [unwired: 1 in, 1 out]
        n231 = call-poly "Enqueue Message.vi"("Priority Message? (F)"=TRUE, "Message"="Exit", "Message Queue"=w715) -> ("error out"=w714:errorcluster, "dup Message Queue"=w713:refnum<queue>)  [unwired: 7 in]
      }
      event "Shoot": Value Change {
        n232 = event-data() -> ()  [unwired: 1 in, 1 out]
        n233 = call-poly "Enqueue Message.vi"("Message"="Shoot", "Message Queue"=w719) -> ("error out"=w716:errorcluster, "dup Message Queue"=w718:refnum<queue>)  [unwired: 8 in]
      }
      event "Start Loop": Value Change {
        n234 = event-data() -> ()  [unwired: 1 in, 1 out]
        n235 = call-poly "Enqueue Message.vi"("Message"="Start Loop", "Message Queue"=w723) -> ("error out"=w720:errorcluster, "dup Message Queue"=w722:refnum<queue>)  [unwired: 8 in]
      }
      event "Sequence Length (ms)": Value Change {
        n236 = event-data() -> ()  [unwired: 1 in, 1 out]
        n237 = To Variant(anything="Sequence Length (ms)") -> (Variant=w724:variant)
        n238 = call-poly "Enqueue Message.vi"("Message Data"=w724, "Message"="UpdateSequenceLength", "Message Queue"=w729) -> ("error out"=w726:errorcluster, "dup Message Queue"=w728:refnum<queue>)  [unwired: 7 in]
      }
      event User Event {
        # "The Message Handling Loop processed an \"Exit\" message, which fired this event to stop the Event Handling Loop."
        n239 = event-data() -> ()  [unwired: 1 in, 4 out]
      }
      event User Event {
        # "It is. You can rename and use this event for something else"
        # "Maybe this should rather go into the \ntarget device consumer loop to detach a message\nto the logging consumer loop"
        n240 = event-data() -> ()  [unwired: 1 in, 4 out]
      }
    }
    n241 = call "Error Handler - Event Handling Loop.vi"("error in (no error)"=w682, "Message Queue"=w680) -> ("dup error in"=w679:errorcluster)  [unwired: 8 in, 1 out]
  }
  n242 = Unregister For Events(event registration refnum=w15, error in=w22) -> (error out=w24:errorcluster)
  n243 = Merge Errors(w24, w29) -> (w26:errorcluster)
  n244 = call "Destroy User Events.vi"("error in (no error)"=w26, "User Events"=w25) -> ("error out"=w7:errorcluster)  [unwired: 9 in]
  n245 = Merge Errors(w7, w3, w2, w1) -> (w4:errorcluster)
  n246 = call "Destroy All Message Queues.vi"("error in (no error)"=w4, "Message Queues"=w6) -> ("error out"=w5:errorcluster)  [unwired: 9 in]
  n247 = disable-structure shown="Default" {
    disable-tunnel: w5 -> [_ _]
    frame condition #0 (active) {
    }
    frame condition #1 {
      # "Call Quit LabVIEW if running as a built application."
      n248 = Quit LabVIEW() -> ()  [unwired: 1 in]
    }
  }
